vi "Module TypeDef.vi"(8 "error in (no error)":errorcluster, 11 "Module in":T1) -> (0 "error out":errorcluster, 3 "Module":T2)   [LabVIEW 2022 SP3, in "Core.lvlib"]
uses:
  Core.lvlib
  Controls/Module.ctl
  Controls/Module Instance.ctl
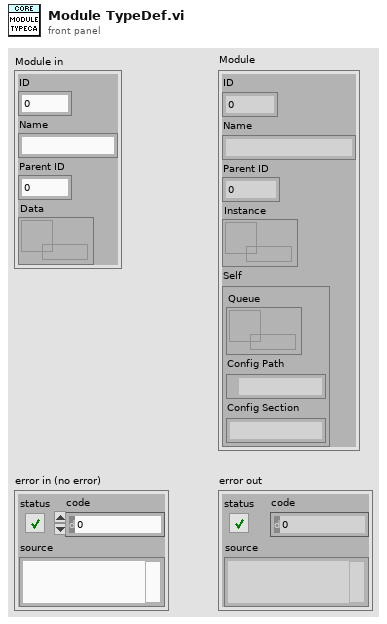
[diagram p1: front panel]
types:
  T1 = cluster{"ID":i32, "Name":string, "Parent ID":i32, "Data":refnum<data-value>}
  T2 = typedef "Core.lvlib/Module.ctl" = cluster{"ID":i32, "Name":string, "Parent ID":i32, "Instance":refnum<data-value>, "Self":T3}
  T3 = typedef "Core.lvlib/Module Instance.ctl" = cluster{"Queue":refnum<queue>, "Config Path":path, "Config Section":string}
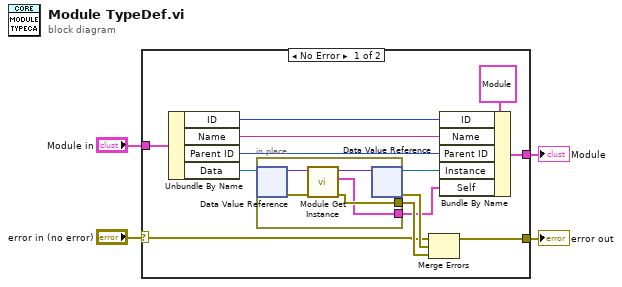
[diagram p0: block diagram]
diagram:
  n1 = case shown="No Error" "error in (no error)" {
    selector: "error in (no error)" -> [w7 w23]
    tunnel: [w16 _] -> w4
    tunnel: "Module in" -> [w15 _]
    tunnel: [w6 w23] -> w1
    frame No Error {
      n2 = Unbundle By Name(w15) -> ("ID"=w14:i32, "Name"=w13:string, "Parent ID"=w12:i32, "Data"=w11:refnum<data-value>)
      n3 = in-place {
        in-place-border: [w19] -> w8
        in-place-border: [w18] -> w5
        n4 = in-place-dvr #1(w11) -> (w22:variant, w21:errorcluster)
        n5 = call "Module Get Instance.vi"("error in (no error)"=w21, "Self in"=w22) -> ("error out"=w19:errorcluster, "Instance"=w18:T3, "Self out"=w20:variant)  [unwired: 7 in]
        n6 = in-place-dvr #1(w20) -> (w10:refnum<data-value>, w9:errorcluster)
      }
      n7 = Merge Errors(w7, w9, w8) -> (w6:errorcluster)
      n8 = Bundle By Name(cluster=T2 {"ID"=0, "Name"="", "Parent ID"=0, "Instance"=refnum, "Self"={"Queue"=refnum, "Config Path"=path "", "Config Section"=""}} ("Module"), "ID"=w14, "Name"=w13, "Parent ID"=w12, "Instance"=w10, "Self"=w5) -> (w16:T2)
    }
    frame Error {
    }
  }
  "Module" <- w4
  "error out" <- w1
